vi "Is Open.vi"(8 "error in (no error)":errorcluster, 11 "VisaResource in":refnum<class "VisaResource.lvclass">) -> (0 "error out":errorcluster, 2 "Is Open":bool, 3 "VisaResource out":refnum<class "VisaResource.lvclass">)   [LabVIEW 2020, in "PicoG-Core.lvlib" / "VisaResource.lvclass"]
uses:
  VisaResource.lvclass
  VisaResource.lvclass/VisaResource.ctl
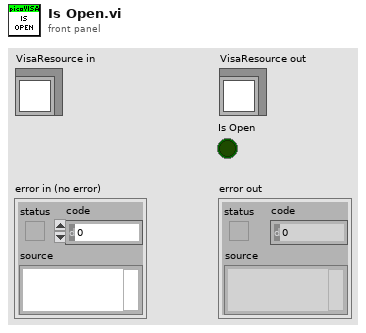
[diagram p1: front panel]
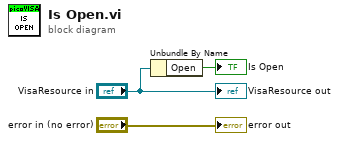
[diagram p0: block diagram]
diagram:
  n1 = Unbundle By Name("VisaResource in") -> ("Open"=→"Is Open":bool)
  "error out" <- "error in (no error)"
  "VisaResource out" <- "VisaResource in"
